vi "FrontPanelOpen.vi"(4 "State":T1(ring)=enum."Standard", 6 "Activate?":bool=TRUE, 8 "error in (no error)":errorcluster, 10 "VI Path":path, 11 "VI in":refnum<vi>) -> (0 "error out":errorcluster, 3 "VI out":refnum<vi>)   [LabVIEW 2013]
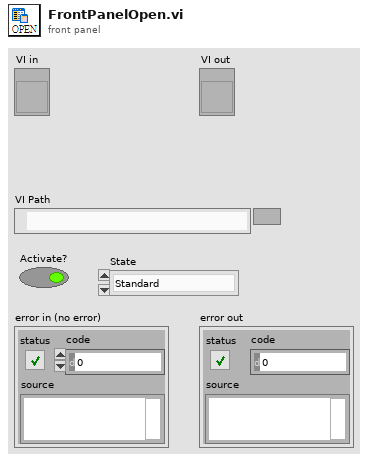
[diagram p1: front panel]
types:
  T1 = enum32{"Invalid", "Standard", "Closed", "Hidden", "Minimized", "Maximized"}
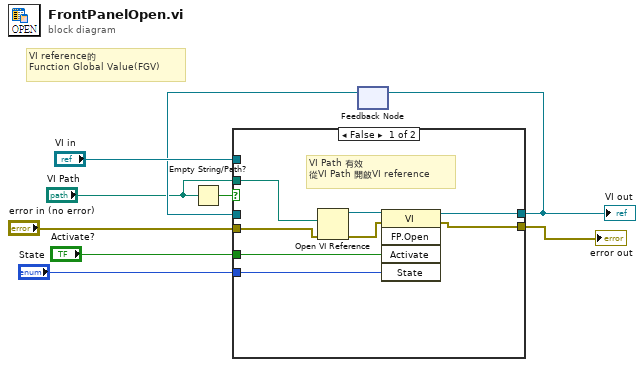
[diagram p0: block diagram]
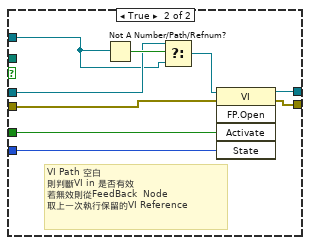
[diagram p2: hidden frame]
diagram:
  # "VI reference的\nFunction Global Value(FGV)"
  n1 = Empty String/Path?(string/path="VI Path") -> (empty?=w7:bool)
  n2 = feedback #1() -> (w8:refnum<vi>)  [unwired: 1 in]
  n3 = case shown="False" w7 {
    tunnel: "Activate?" -> [w17 w23]
    tunnel: "State" -> [w16 w22]
    tunnel: [w15 w26] -> w6
    tunnel: [w14 w25] -> w4
    tunnel: "error in (no error)" -> [w11 w24]
    tunnel: "VI Path" -> [w10 _]
    tunnel: w8 -> [_ w20]
    tunnel: "VI in" -> [_ w18]
    frame False {
      # "VI Path 有效\n從VI Path 開啟VI reference"
      n4 = Open VI Reference(vi path=w10, error in (no error)=w11) -> (vi reference=w13:refnum<vi>, error out=w12:errorcluster)  [unwired: 4 in]
      n5 = invoke class="VI" method="FP.Open"(reference=w13, error in=w12, "Activate"=w17, "State"=w16) -> (reference out=w15:refnum<vi>, error out=w14:errorcluster)  [unwired: 1 in, 3 out]
    }
    frame True {
      # "VI Path 空白\n則判斷VI in 是否有效\n若無效則從FeedBack  Node\n取上一次執行保留的VI Reference"
      n6 = Not A Number/Path/Refnum?(number/path/refnum=w18) -> (NaN/Path/Refnum?=w21:bool)
      n7 = Select(t=w20, s=w21, f=w18) -> (s? t:f=w19:refnum<vi>)
      n8 = invoke class="VI" method="FP.Open"(reference=w19, error in=w24, "Activate"=w23, "State"=w22) -> (reference out=w26:refnum<vi>, error out=w25:errorcluster)  [unwired: 1 in, 3 out]
    }
  }
  "VI out" <- w6
  "error out" <- w4
  n9 = feedback-in #1(w6) -> ()
